vi "Server.vi"() -> ()   [LabVIEW 2013]
uses:
  <vilib>/OPCUA/NI OPC UA Server.lvlib
  OPCUA XML/CreateOPCUAServerAuto.lvlib
panel:
  out "xml path":path
  out "trusted client certfications":path[](array[path])
  out "Parse Errors":string
  out "ready":bool
  out "server endpoint URL":string
  in  "show structure":bool
  out "error out":errorcluster
  in  "stop":bool
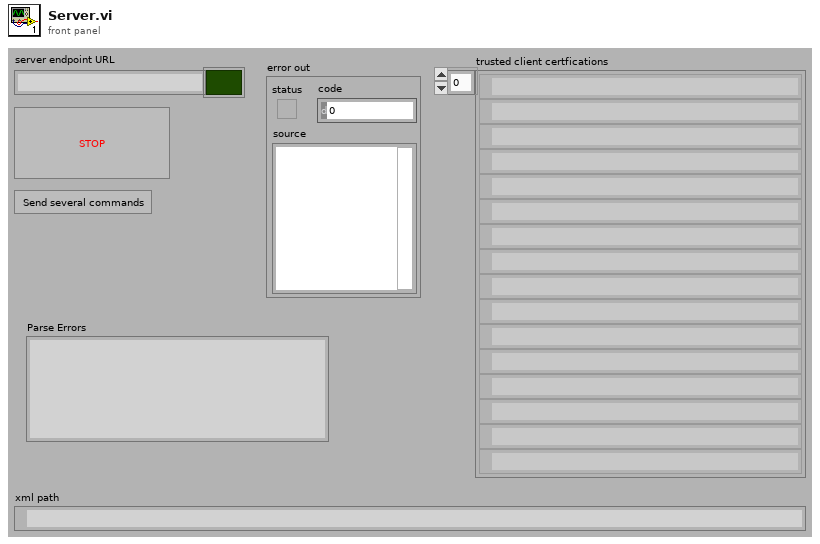
[diagram p1: front panel]
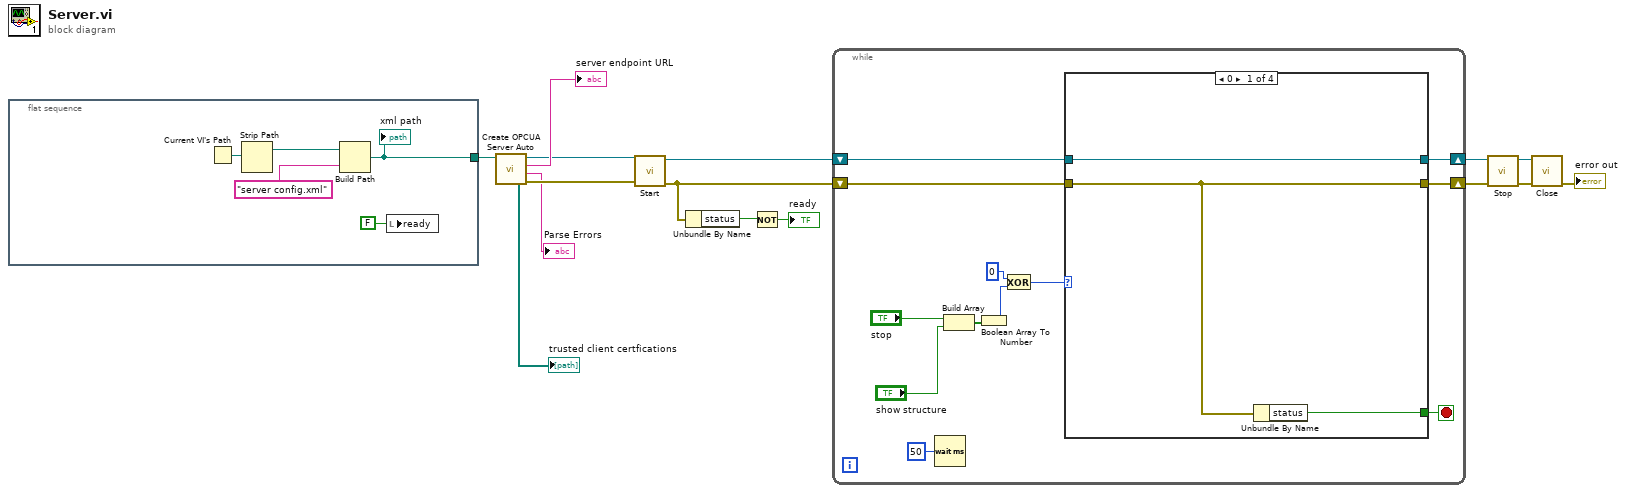
[diagram p0: block diagram]
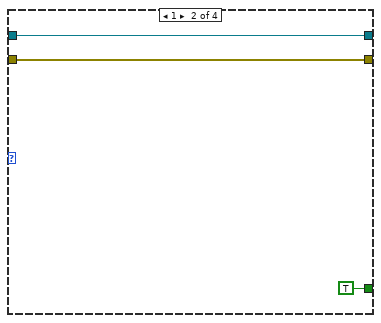
[diagram p2: hidden frame]
diagram:
  n1 = flat-sequence {
    tunnel: [w16] -> w1
    frame #0 {
      n2 = Current VI's Path() -> (path=w19:path)
      n3 = Strip Path(path=w19) -> (stripped path=w18:path)  [unwired: 1 out]
      n4 = Build Path(base path=w18, name or relative path="server config.xml") -> (appended path=w16:path)
      "xml path" <- w16
      n5 = local write "ready"(FALSE) -> ()
    }
  }
  n6 = call "Create OPCUA Server Auto.vi"("XML config File Path"=w1) -> ("Error Out"=w4:errorcluster, "Parse Errors"=→"Parse Errors":string, "server endpoint URL"=→"server endpoint URL":string, "OPC UA server refnum out"=w5:refnum<k21>, "trusted client certfications"=→"trusted client certfications":path[])  [unwired: 6 in]
  n7 = call <vilib>:"Start.vi"("error in (no error)"=w4, "OPC UA server refnum in"=w5) -> ("error out"=w8:errorcluster, "OPC UA server refnum out"=w15:refnum<k21>)  [unwired: 8 in]
  n8 = Unbundle By Name(w8) -> ("status"=w7:bool)
  n9 = Not(x=w7) -> (.not. x?=→"ready":bool)
  n10 = while {
    shift-right: [w26] -> w12
    shift-left: w15 -> [w25]
    shift-right: [w23] -> w10
    shift-left: w8 -> [w24]
    stop <- w22 stop-if-true
    n11 = Wait (ms)(milliseconds to wait=u32 50) -> ()  [unwired: 1 out]
    n12 = Build Array("stop", "show structure") -> (w29:bool[])
    n13 = Boolean Array To Number(Boolean array=w29) -> (number=w21:u32)
    n14 = Exclusive Or(1:w21, 2:u32 0) -> (0:w27:u32)
    n15 = case shown="0" w27 {
      tunnel: [w35 w38 w40 w42] -> w26
      tunnel: w25 -> [w35 w38 w40 w42]
      tunnel: w24 -> [w33 w37 w39 w41]
      tunnel: [w33 w37 w39 w41] -> w23
      tunnel: [w34 TRUE _ _] -> w22
      frame 0 {
        n16 = Unbundle By Name(w33) -> ("status"=w34:bool)
      }
      frame 1 {
      }
      frame 2 {
      }
      frame Default {
      }
    }
  }
  n17 = call <vilib>:"Stop.vi"("error in (no error)"=w10, "OPC UA server refnum in"=w12) -> ("error out"=w9:errorcluster, "OPC UA server refnum out"=w11:refnum<k21>)  [unwired: 8 in]
  n18 = call <vilib>:"Close.vi"("error in (no error)"=w9, "OPC UA server refnum in"=w11) -> ("error out"=→"error out":errorcluster)  [unwired: 9 in]
